vi "XML Get Node Data by Variant.vi"(4 "level":i32, 5 "element id":i32, 6 "Attribute?(F=Entity)":bool, 7 "Type Formatting":T1, 8 "error in (no error)":errorcluster, 10 "Variant in (type and name)":variant, 11 "xml":T3) -> (0 "error out":errorcluster, 2 "Variant out":variant)   [LabVIEW 2011]
uses:
  Fast Parser/XML Structure - Cluster.ctl
  Fast Parser/XML Tag Type - Enum.ctl
  Options API/Private/EasyXML Options - Type Formatting Cluster.ctl
  Type Defs/Formatting Data Type -- Enum.ctl
  Get Node Data.vi
  Poly Members/Get Node Data (EXT).vi
panel:
  # "Copyright © 2006 James Kring, Inc. All rights reserved.\n\nAuthor: Jim Kring <jim.kring@jameskring.com>\n\nThis library is provided \"AS IS\" , WITHOUT WARRANTIES OR \nCONDITIONS OF ANY KIND, either express or implied.\n\nJames Kring, Inc. -- http://www.jameskring.com"
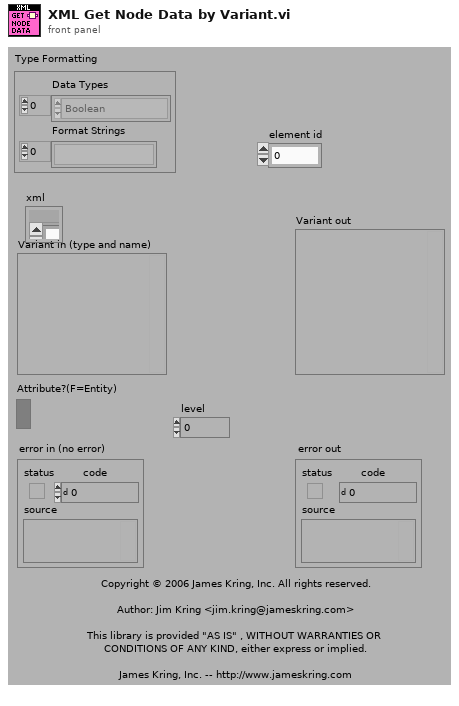
[diagram p1: front panel]
types:
  T1 = typedef "EasyXML Options - Type Formatting Cluster.ctl" = cluster{"Data Types":T2[], "Format Strings":string[]}
  T2 = typedef "Formatting Data Type -- Enum.ctl" = enum16{"<unknown>", "Cluster", "Array", "String", "Path", "Boolean", "Time Stamp", "Enum", "Numeric - EXT", "Numeric - DBL", "Numeric - SGL", "Numeric - I64", "Numeric - I32", "Numeric - I16", "Numeric - I8", "Numeric - U64", "Numeric - U32", "Numeric - U16", "Numeric - U8", "Numeric - CXT", "Numeric - CDB", "Numeric - CSG", "VISA Resource"}
  T3 = typedef "XML Structure - Cluster.ctl" = cluster{"tags":string[], "tag names":string[], "tag type":T4[], "offset":i32[], "close tag index":i32[], "xml":string, "Children":cluster{"children":i32[]}[], "parent index":i32[]}
  T4 = typedef "XML Tag Type - Enum.ctl" = enum16{"start tag", "empty tag", "end tag"}
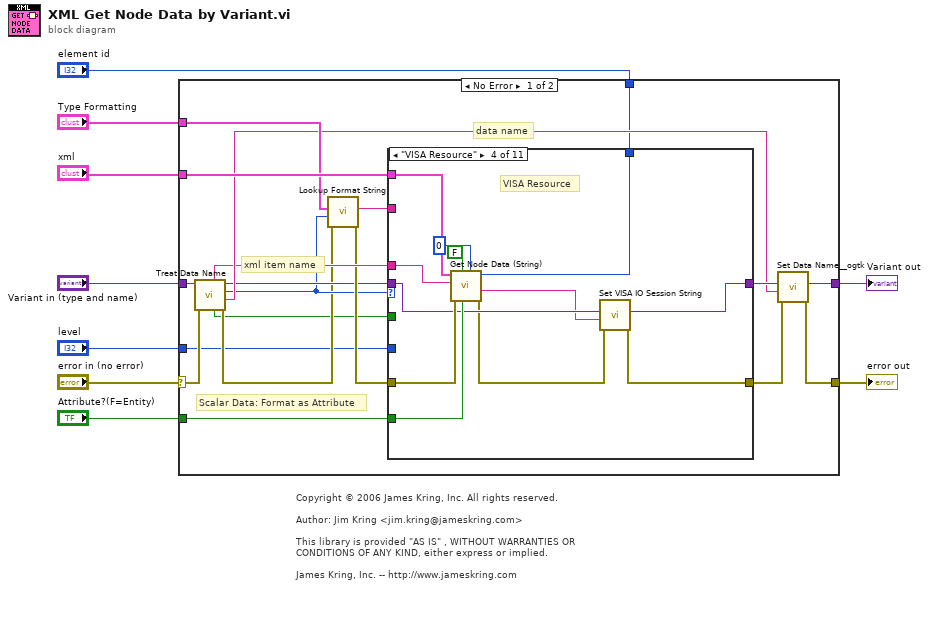
[diagram p0: block diagram]
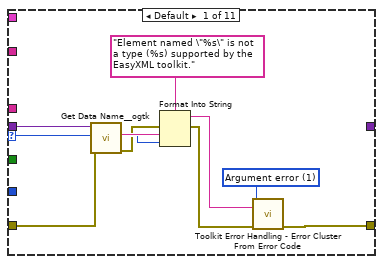
[diagram p2: hidden frame]
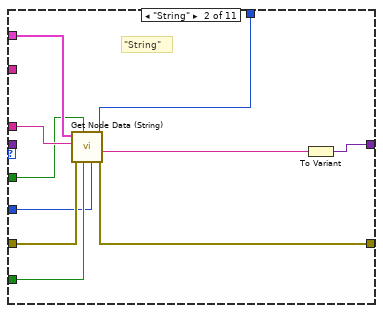
[diagram p3: hidden frame]
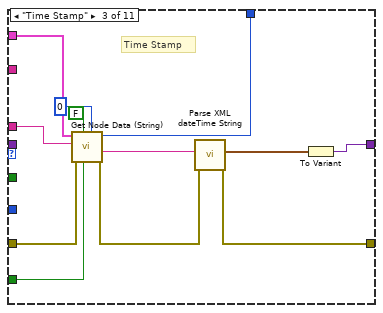
[diagram p4: hidden frame]
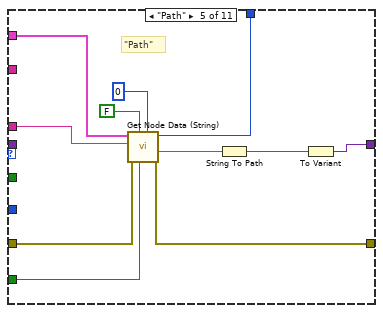
[diagram p5: hidden frame]
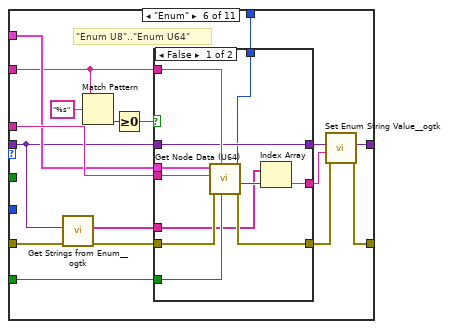
[diagram p6: hidden frame]
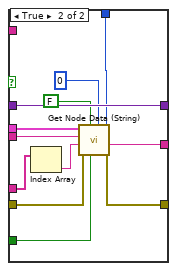
[diagram p7: hidden frame]
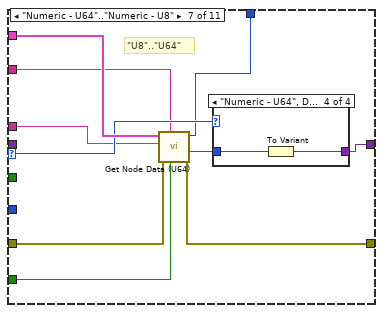
[diagram p8: hidden frame]
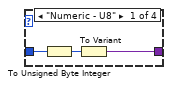
[diagram p9: hidden frame]
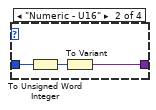
[diagram p10: hidden frame]
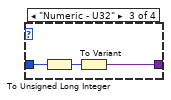
[diagram p11: hidden frame]
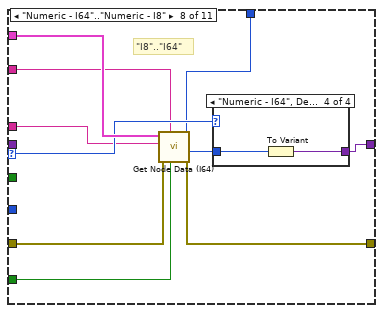
[diagram p12: hidden frame]
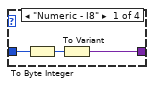
[diagram p13: hidden frame]
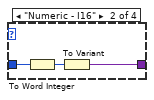
[diagram p14: hidden frame]
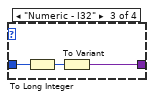
[diagram p15: hidden frame]
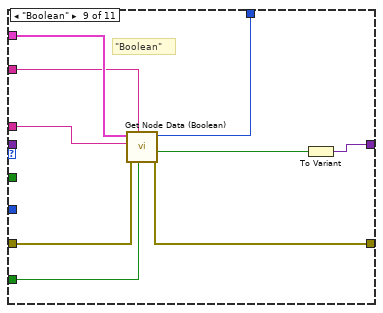
[diagram p16: hidden frame]
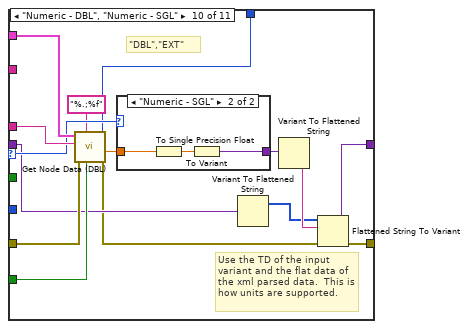
[diagram p17: hidden frame]
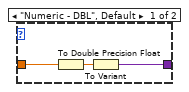
[diagram p18: hidden frame]
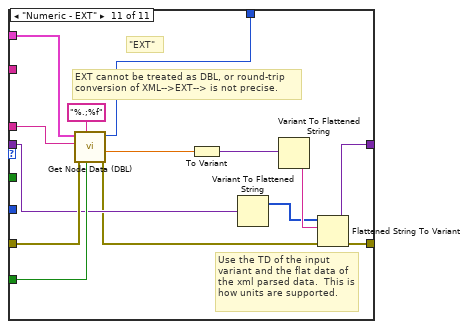
[diagram p19: hidden frame]
diagram:
  # "Copyright © 2006 James Kring, Inc. All rights reserved.\n\nAuthor: Jim Kring <jim.kring@jameskring.com>\n\nThis library is provided \"AS IS\" , WITHOUT WARRANTIES OR \nCONDITIONS OF ANY KIND, either express or implied.\n\nJames Kring, Inc. -- http://www.jameskring.com"
  n1 = case shown="No Error" "error in (no error)" {
    selector: "error in (no error)" -> [w15 w211]
    tunnel: "Variant in (type and name)" -> [w16 w210]
    tunnel: "xml" -> [w28 _]
    tunnel: [w26 w210] -> w7
    tunnel: [w25 w211] -> w8
    tunnel: "Type Formatting" -> [w22 _]
    tunnel: "Attribute?(F=Entity)" -> [w23 _]
    tunnel: "level" -> [w11 _]
    tunnel: "element id" -> [w10 _]
    frame No Error {
      # "xml item name"
      # "data name"
      # "Scalar Data: Format as Attribute"
      n2 = call "Treat Data Name.vi"("error in (no error)"=w15, "Data"=w16) -> ("error out"=w13:errorcluster, "untreated Data Name"=w20:string, "EasyXML Type"=w14:T2, "dup Data"=w17:variant, "contains raw xml?"=w12:bool, "treated xml name"=w19:string)  [unwired: 3 in, 1 out]
      n3 = call "Lookup Format String.vi"("error in"=w13, "element"=w14, "Type Formatting"=w22) -> ("error out"=w18:errorcluster, "Format String"=w21:string)  [unwired: 5 in, 2 out]
      n4 = case shown="\"VISA Resource\"" w14 {
        selector: w14 -> [w33 _ _ _ _ _ w128 w149 _ w184 _]
        tunnel: w28 -> [_ w48 w60 w72 w83 w97 w133 w154 w174 w189 w209]
        tunnel: w18 -> [w32 w47 w59 w71 w82 w100 w132 w153 w173 w188 w208]
        tunnel: [w29 w46 w54 w63 w81 w88 w131 w152 w172 w179 w201] -> w24
        tunnel: [_ w44 w58 w64 w79 w89 w130 w151 w171 w178 w200] -> w27
        tunnel: w17 -> [w34 _ _ w65 _ w92 _ _ _ w183 w205]
        tunnel: w21 -> [_ _ _ _ _ w91 w125 w146 w167 _ _]
        tunnel: w23 -> [_ w42 w56 w69 w77 w98 w127 w148 w168 w187 w207]
        tunnel: w19 -> [_ w43 w57 w70 w78 w99 w126 w147 w169 w186 w206]
        tunnel: w12 -> [_ w41 _ _ _ _ _ _ _ _ _]
        tunnel: w11 -> [_ w39 _ _ _ _ _ _ _ _ _]
        tunnel: w10 -> [_ w40 w49 w66 w73 w84 w124 w145 w166 w176 w198]
        frame Default {
          w36 = 1 items=["No error", "Argument error", "Memory is full", "Out of zone", "End of file", "File already open", "Generic file I/O error", "File not found", "File permission error", "Disk is full", "Duplicate path", "Too many files open", "System feature not enabled", "Resource file not found", "Cannot add resource", "Resource not found", "Image not found", "Image memory error", "Pen does not exist", "Config type invalid", "Config token not found", "Config parse error", "Config memory error", "Bad external code format", "Bad external code offset", "External code not present", "Null window", "Destroy window error", "Null menu", "Print aborted", "Bad print record", "Print driver error", "Windows error during printing", "Memory error during printing", "Print dialog error", "Generic print error", "Invalid device refnum", "Device not found", "Device parameter error", "Device unit error", "Cannot open device", "Device call aborted", "Generic error", "Cancelled by user", "Object ID too low", "Object ID too high", "Object not in heap", "Unknown heap", "Unknown object (invalid DefProc)", "Unknown object (DefProc not in table)", "Message out of range", "Invalid (null) method", "Unknown message", "Manager call not supported", "Bad address", "Network operation in progress", "Network operation timed out", "Connection is busy", "Network attribute not supported", "Network error", "Address in use", "System out of memory", "Connection aborted", "Connection refused", "Not connected", "Already connected", "Connection closed", "Initialization error (interapplication manager)", "Bad occurrence", "Wait on unbound occurrence handler", "Occurrence queue overflow", "Datalog type conflict", "Unused", "Unrecognized type (interapplication manager)", "Memory corrupt", "Failed to make temporary DLL", "Old CIN version", "Drag socket not found", "Failed to load drop-object", "Failed to register OLE object", "Failed to release OLE object", "Format specifier type mismatch", "Unknown format specifier", "Too few format specifiers", "Too many format specifiers", "Scan failed", "Newer CIN version", "Error converting to variant", "Runtime menu error", "Password tampered", "Variant attribute not found", "Incompatible variant data type", "Event data is not available", "Event Store is not present", "Occurrence is not found", "Event Queue is not created", "Event info is not available", "Refnum passed is NULL", "Error retrieving Class GUID", "Error retrieving CoClass GUID", "Error retrieving TypeLib GUID.", "Bad built application magic bytes.", "Specific driver is different from the specific driver associated with the Logical Name.", "There is no session opened to the class driver.", "Max Error", "MAX - Error with config objects", "MAX - Error loading configuration", "MAX - Group not supported"]
          n5 = call <userlib>:"Get Data Name__ogtk.vi"("error in (no error)"=w32, "Data"=w34) -> ("error out"=w31:errorcluster, "Data Name"=w38:string)  [unwired: 7 in, 1 out]
          n6 = Format Into String(format string="Element named \"%s\" is not a type (%s) supported by the EasyXML toolkit." ("Format String"), error in=w31, w38, w33) -> (resulting string=w35:string, error out=w30:errorcluster)  [unwired: 1 in]
          n7 = call "Toolkit Error Handling - Error Cluster From Error Code.vi"("error in"=w30, "error message (\"\")"=w35, "error code (0)"=w36) -> ("error out"=w29:errorcluster)  [unwired: 6 in]
        }
        frame "String" {
          # "\"String\""
          n8 = call-poly "Get Node Data (String).vi"("element id"=w40, "level"=w39, "Attribute? (F=Entity)"=w42, "contains raw xml"=w41, "error in (no error)"=w47, "Attribute Name"=w43, "xml"=w48) -> ("error out"=w46:errorcluster, "Data Value"=w45:string)  [unwired: 2 in, 1 out]
          n9 = To Variant(anything=w45) -> (Variant=w44:variant)
        }
        frame "Time Stamp" {
          # "Time Stamp"
          n10 = call-poly "Get Node Data (String).vi"("element id"=w49, "level"=0, "Attribute? (F=Entity)"=w56, "contains raw xml"=FALSE, "error in (no error)"=w59, "Attribute Name"=w57, "xml"=w60) -> ("error out"=w55:errorcluster, "Data Value"=w53:string)  [unwired: 2 in, 1 out]
          n11 = call "Parse XML dateTime String.vi"("error in (no error)"=w55, "xml dateTime string"=w53) -> ("error out"=w54:errorcluster, "Time Stamp"=w52:timestamp)  [unwired: 8 in]
          n12 = To Variant(anything=w52) -> (Variant=w58:variant)
        }
        frame "VISA Resource" {
          # "VISA Resource"
          n13 = call-poly "Get Node Data (String).vi"("element id"=w66, "level"=0, "Attribute? (F=Entity)"=w69, "contains raw xml"=FALSE, "error in (no error)"=w71, "Attribute Name"=w70, "xml"=w72) -> ("error out"=w62:errorcluster, "Data Value"=w61:string)  [unwired: 2 in, 1 out]
          n14 = call "Set VISA IO Session String.vi"("error in (no error)"=w62, "String"=w61, "Variant in (type and name)"=w65) -> ("error out"=w63:errorcluster, "Variant"=w64:variant)  [unwired: 7 in]
        }
        frame "Path" {
          # "\"Path\""
          n15 = call-poly "Get Node Data (String).vi"("element id"=w73, "level"=0, "Attribute? (F=Entity)"=w77, "contains raw xml"=FALSE, "error in (no error)"=w82, "Attribute Name"=w78, "xml"=w83) -> ("error out"=w81:errorcluster, "Data Value"=w80:string)  [unwired: 2 in, 1 out]
          n16 = String To Path(string=w80) -> (path=w76:path)
          n17 = To Variant(anything=w76) -> (Variant=w79:variant)
        }
        frame "Enum" {
          # "\"Enum U8\"..\"Enum U64\""
          n18 = call <userlib>:"Get Strings from Enum__ogtk.vi"("error in (no error)"=w100, "Enum"=w92) -> ("error out"=w95:errorcluster, "Enum Strings"=w85:string[])  [unwired: 6 in, 2 out]
          n19 = Match Pattern(string=w91, regular expression="%s") -> (offset past match=w94:i32)  [unwired: 1 in, 3 out]
          n20 = Greater Or Equal To 0?(x=w94) -> (x >= 0?=w93:bool)
          n21 = case shown="False" w93 {
            tunnel: w99 -> [w109 w123]
            tunnel: w98 -> [w107 w122]
            tunnel: [w106 w117] -> w87
            tunnel: w97 -> [w110 w121]
            tunnel: w95 -> [w108 w120]
            tunnel: w92 -> [w102 w119]
            tunnel: [w102 w119] -> w90
            tunnel: w91 -> [w111 _]
            tunnel: [w103 w118] -> w86
            tunnel: w85 -> [w104 w116]
            tunnel: w84 -> [w101 w112]
            frame False {
              n22 = call-poly "Get Node Data (U64).vi"("element id"=w101, "Attribute?(F=Entity)"=w107, "format string (%d)"=w111, "error in"=w108, "Attribute Name"=w109, "xml"=w110) -> ("error out"=w106:errorcluster, "Data Value"=w105:u64)  [unwired: 3 in, 1 out]
              n23 = Index Array(array=w104, index=w105) -> (element=w103:string)
            }
            frame True {
              n24 = Index Array(array=w116) -> (element=w115:string)  [unwired: 1 in]
              n25 = call-poly "Get Node Data (String).vi"("element id"=w112, "level"=0, "Attribute? (F=Entity)"=w122, "contains raw xml"=FALSE, "error in (no error)"=w120, "Default Value (\"\")"=w115, "Attribute Name"=w123, "xml"=w121) -> ("error out"=w117:errorcluster, "Data Value"=w118:string)  [unwired: 1 in, 1 out]
            }
          }
          n26 = call <userlib>:"Set Enum String Value__ogtk.vi"("error in (no error)"=w87, "String Value"=w86, "Default Enum Value"=w90) -> ("error out"=w88:errorcluster, "Enum"=w89:variant)  [unwired: 7 in]
        }
        frame "Numeric - U64".."Numeric - U8" {
          # "\"U8\"..\"U64\""
          n27 = call-poly "Get Node Data (U64).vi"("element id"=w124, "Attribute?(F=Entity)"=w127, "format string (%d)"=w125, "error in"=w132, "Attribute Name"=w126, "xml"=w133) -> ("error out"=w131:errorcluster, "Data Value"=w129:u64)  [unwired: 3 in, 1 out]
          n28 = case shown="\"Numeric - U64\", Default" w128 {
            tunnel: w129 -> [w136 w139 w142 w143]
            tunnel: [w135 w138 w141 w144] -> w130
            frame "Numeric - U8" {
              n29 = To Unsigned Byte Integer(number=w136) -> (unsigned 8bit integer=w134:u8)
              n30 = To Variant(anything=w134) -> (Variant=w135:variant)
            }
            frame "Numeric - U16" {
              n31 = To Unsigned Word Integer(number=w139) -> (unsigned 16bit integer=w137:u16)
              n32 = To Variant(anything=w137) -> (Variant=w138:variant)
            }
            frame "Numeric - U32" {
              n33 = To Unsigned Long Integer(number=w142) -> (unsigned 32bit integer=w140:u32)
              n34 = To Variant(anything=w140) -> (Variant=w141:variant)
            }
            frame "Numeric - U64", Default {
              n35 = To Variant(anything=w143) -> (Variant=w144:variant)
            }
          }
        }
        frame "Numeric - I64".."Numeric - I8" {
          # "\"I8\"..\"I64\""
          n36 = call-poly "Get Node Data (I64).vi"("element id"=w145, "Attribute?(F=Entity)"=w148, "format string (%d)"=w146, "error in"=w153, "Attribute Name"=w147, "xml"=w154) -> ("error out"=w152:errorcluster, "Data Value"=w150:i64)  [unwired: 3 in, 1 out]
          n37 = case shown="\"Numeric - I64\", Default" w149 {
            tunnel: w150 -> [w157 w160 w163 w164]
            tunnel: [w156 w159 w162 w165] -> w151
            frame "Numeric - I8" {
              n38 = To Byte Integer(number=w157) -> (8bit integer=w155:i8)
              n39 = To Variant(anything=w155) -> (Variant=w156:variant)
            }
            frame "Numeric - I16" {
              n40 = To Word Integer(number=w160) -> (16bit integer=w158:i16)
              n41 = To Variant(anything=w158) -> (Variant=w159:variant)
            }
            frame "Numeric - I32" {
              n42 = To Long Integer(number=w163) -> (32bit integer=w161:i32)
              n43 = To Variant(anything=w161) -> (Variant=w162:variant)
            }
            frame "Numeric - I64", Default {
              n44 = To Variant(anything=w164) -> (Variant=w165:variant)
            }
          }
        }
        frame "Boolean" {
          # "\"Boolean\""
          n45 = call-poly "Get Node Data (Boolean).vi"("element id"=w166, "Attribute?(F=Entity)"=w168, "format string (%d)"=w167, "error in"=w173, "Attribute Name"=w169, "xml"=w174) -> ("error out"=w172:errorcluster, "Data Value"=w170:bool)  [unwired: 3 in, 1 out]
          n46 = To Variant(anything=w170) -> (Variant=w171:variant)
        }
        frame "Numeric - DBL", "Numeric - SGL" {
          # "Use the TD of the input variant and the flat data of the xml parsed data.  This is how units are supported."
          # "\"DBL\",\"EXT\""
          n47 = call-poly "Get Node Data (DBL).vi"("element id"=w176, "Attribute?(F=Entity)"=w187, "format string"="%.;%f", "error in"=w188, "Attribute Name"=w186, "xml"=w189) -> ("error out"=w180:errorcluster, "Attribute Value"=w185:dbl)  [unwired: 3 in, 1 out]
          n48 = case shown="\"Numeric - SGL\"" w184 {
            tunnel: w185 -> [w192 w195]
            tunnel: [w191 w194] -> w177
            frame "Numeric - DBL", Default {
              n49 = To Double Precision Float(number=w192) -> (double precision float=w190:dbl)
              n50 = To Variant(anything=w190) -> (Variant=w191:variant)
            }
            frame "Numeric - SGL" {
              n51 = To Single Precision Float(number=w195) -> (single precision float=w193:sgl)
              n52 = To Variant(anything=w193) -> (Variant=w194:variant)
            }
          }
          n53 = Variant To Flattened String(Variant=w183) -> (1:w181:i16[])  [unwired: 1 out]
          n54 = Variant To Flattened String(Variant=w177) -> (data string=w182:string)  [unwired: 1 out]
          n55 = Flattened String To Variant(4:w180, 6:w182, 7:w181) -> (0:w179:errorcluster, 3:w178:variant)
        }
        frame "Numeric - EXT" {
          # "EXT cannot be treated as DBL, or round-trip conversion of XML-->EXT--> is not precise."
          # "Use the TD of the input variant and the flat data of the xml parsed data.  This is how units are supported."
          # "\"EXT\""
          n56 = call-poly "Get Node Data (DBL).vi"("element id"=w198, "Attribute?(F=Entity)"=w207, "format string"="%.;%f", "error in"=w208, "Attribute Name"=w206, "xml"=w209) -> ("error out"=w202:errorcluster, "Attribute Value"=w197:ext)  [unwired: 3 in, 1 out]
          n57 = To Variant(anything=w197) -> (Variant=w199:variant)
          n58 = Variant To Flattened String(Variant=w205) -> (1:w203:i16[])  [unwired: 1 out]
          n59 = Variant To Flattened String(Variant=w199) -> (data string=w204:string)  [unwired: 1 out]
          n60 = Flattened String To Variant(4:w202, 6:w204, 7:w203) -> (0:w201:errorcluster, 3:w200:variant)
        }
      }
      n61 = call <userlib>:"Set Data Name__ogtk.vi"("error in (no error)"=w24, "Data Name"=w20, "Data"=w27) -> ("error out"=w25:errorcluster, "Renamed Data"=w26:variant)  [unwired: 7 in]
    }
    frame Error {
    }
  }
  "error out" <- w8
  "Variant out" <- w7
